vi "Build Item to String.vi"(7 "Package Folder":path, 11 "Build Item":T1) -> (3 "String":string)   [LabVIEW 2020, in "neg-pkg.lvlib" / "Package.lvclass"]
uses:
  Package.lvclass
  Build Item.ctl
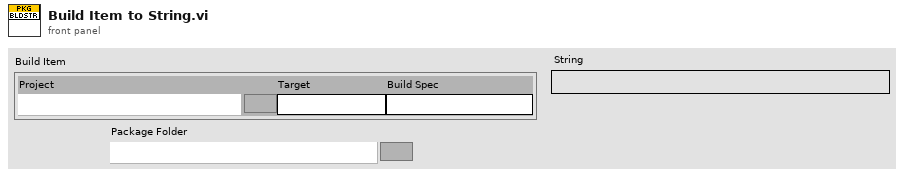
[diagram p1: front panel]
types:
  T1 = typedef "neg-pkg.lvlib/Package.lvclass/Build Item.ctl" = cluster{"Project":path, "Target":string, "Build Spec":string}
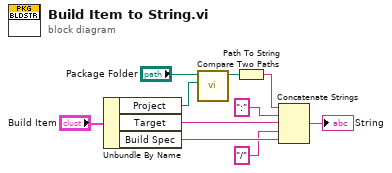
[diagram p0: block diagram]
diagram:
  n1 = Unbundle By Name("Build Item") -> ("Project"=w9:path, "Target"=w5:string, "Build Spec"=w6:string)
  n2 = call <vilib>:"Compare Two Paths.vi"("Path 2"=w9, "Path 1"="Package Folder") -> ("Relative Path from 1 to 2"=w7:path)  [unwired: 6 in, 3 out]
  n3 = Path To String(path=w7) -> (string=w2:string)
  n4 = Concatenate Strings(w2, ":" ("string"), w5, "/" ("string"), w6) -> (→"String":string)
